vi "RX-SIM-SIS-UDP (SubVI).vi"(8 "error in (no error)":errorcluster, 11 "UDP Network Connection in":refnum<k16>) -> (0 "error out":errorcluster, 2 "SIM-SIS-RX-ARRAY":dbl[](array[numeric]), 3 "UDP Network Connection out":refnum<k16>, 4 "SIS-10TI101":dbl, 5 "SIS-10LI202":dbl, 6 "SIS-10AI301":dbl, 7 "SIS-10LI201":dbl)   [LabVIEW 2018]
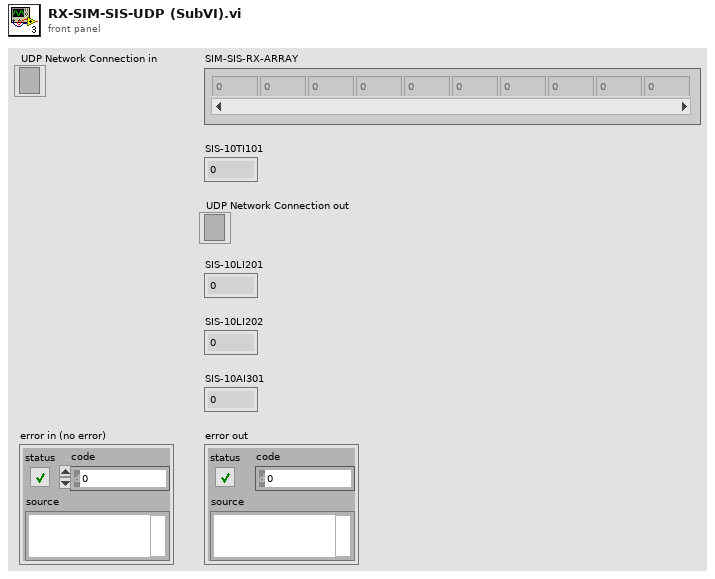
[diagram p1: front panel]
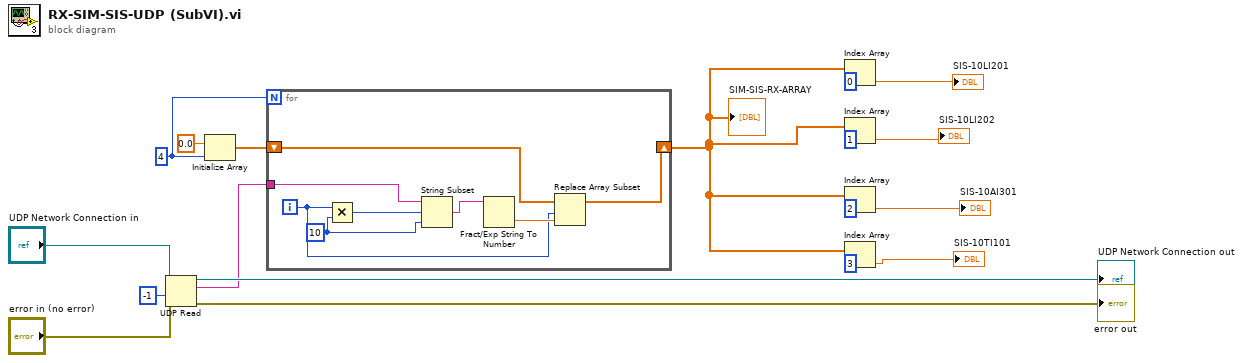
[diagram p0: block diagram]
diagram:
  w8 = 4 ("dimension size")
  n1 = UDP Read(connection ID="UDP Network Connection in", timeout ms (25000)=-1, 8:"error in (no error)") -> (data out=w3:string, error out=→"error out":errorcluster, 3:→"UDP Network Connection out":refnum<k16>)  [unwired: 3 out]
  n2 = Initialize Array(0.0 ("element"), w8) -> (w7:dbl[])
  n3 = for {
    N: w8 -> [_]
    tunnel: w3 -> [w25]
    shift-right: [w21] -> w13
    shift-left: w7 -> [w20]
    i -> [w22]
    w19 = 10 ("y")
    n4 = Multiply(x=w22, y=w19) -> (x*y=w24:i32)
    n5 = String Subset(string=w25, offset (0)=w24, length (rest)=w19) -> (substring=w26:string)
    n6 = Fract/Exp String To Number(string=w26) -> (number=w23:dbl)  [unwired: 3 in, 1 out]
    n7 = Replace Array Subset(array=w20, new element=w23, index=w22) -> (w21:dbl[])
  }
  "SIM-SIS-RX-ARRAY" <- w13
  n8 = Index Array(array=w13, index=0) -> (element=→"SIS-10LI201":dbl)
  n9 = Index Array(array=w13, index=1) -> (element=→"SIS-10LI202":dbl)
  n10 = Index Array(array=w13, index=2) -> (element=→"SIS-10AI301":dbl)
  n11 = Index Array(array=w13, index=3) -> (element=→"SIS-10TI101":dbl)
